vi "SRTS_Set Properties.vi"(8 "error in":errorcluster, 11 "TDMS in":refnum<class "TDMS.lvclass">) -> (0 "error out":errorcluster, 3 "TDMS out":refnum<class "TDMS.lvclass">)   [LabVIEW 2017, in "Report_lib.lvlib" / "TDMS.lvclass"]
uses:
  TDMS.lvclass
  Channels names.ctl
  TDMS.lvclass/TDMS.ctl
panel:
  out "size(s)":i32
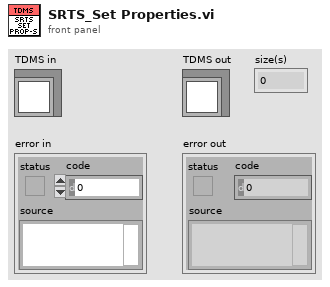
[diagram p1: front panel]
types:
  T1 = typedef "Channels names.ctl" = cluster{"AIM ch.names":string[], "TIM ch.names":string[], "RIM1 ch.names":string[], "RIM2 ch.names":string[], "RIM3 ch.names":string[], "AOM ch.names":string[], "DOM ch.hames":string[]}
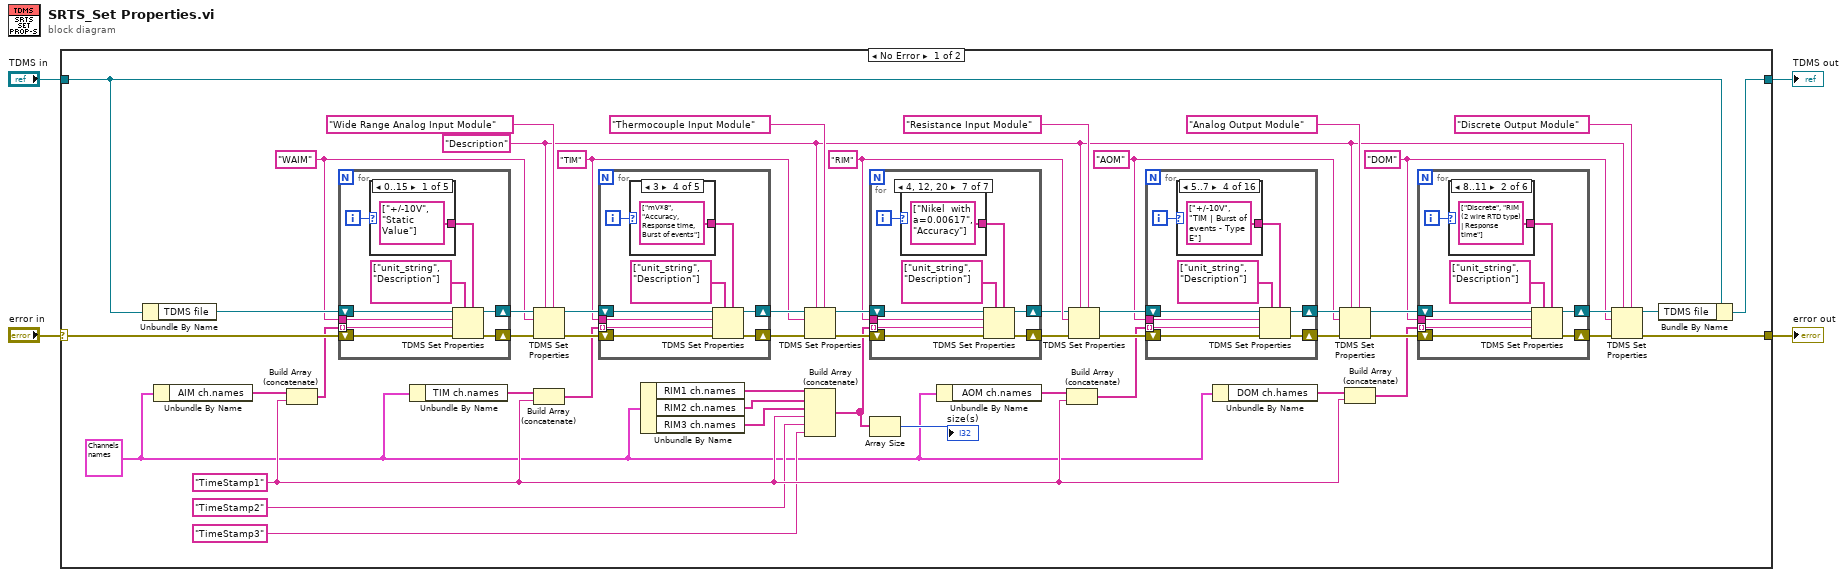
[diagram p0: block diagram]
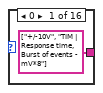
[diagram p2: hidden frame]
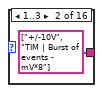
[diagram p3: hidden frame]
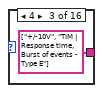
[diagram p4: hidden frame]
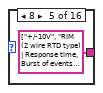
[diagram p5: hidden frame]
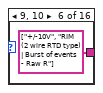
[diagram p6: hidden frame]
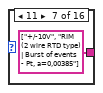
[diagram p7: hidden frame]
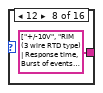
[diagram p8: hidden frame]
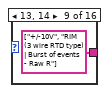
[diagram p9: hidden frame]
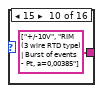
[diagram p10: hidden frame]
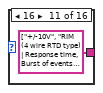
[diagram p11: hidden frame]
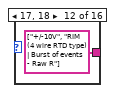
[diagram p12: hidden frame]
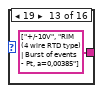
[diagram p13: hidden frame]
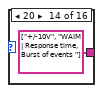
[diagram p14: hidden frame]
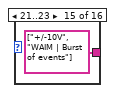
[diagram p15: hidden frame]
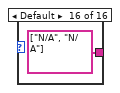
[diagram p16: hidden frame]
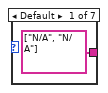
[diagram p17: hidden frame]
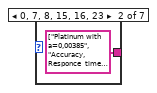
[diagram p18: hidden frame]
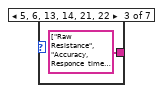
[diagram p19: hidden frame]
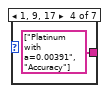
[diagram p20: hidden frame]
diagram:
  n1 = case shown="No Error" "error in" {
    selector: "error in" -> [w48 w142]
    tunnel: [w53 w142] -> w3
    tunnel: [w21 w141] -> w1
    tunnel: "TDMS in" -> [w22 w141]
    frame No Error {
      w5 = T1 {"AIM ch.names"=["05_waim_01ch", "05_waim_02ch", "05_waim_03ch", "05_waim_04ch", "05_waim_05ch", "05_waim_06ch", "05_waim_07ch", "05_waim_08ch", "05_waim_09ch", "05_waim_10ch", "05_waim_11ch", "05_waim_12ch", "05_waim_13ch", "05_waim_14ch", "05_waim_15ch", "05_waim_16ch", "05_waim_17ch", "05_waim_18ch", "05_waim_19ch", "05_waim_20ch", "05_waim_21ch", "05_waim_22ch", "05_waim_23ch", "05_waim_24ch", "05_waim_25ch", "05_waim_26ch", "05_waim_27ch", "05_waim_28ch", "05_waim_29ch", "05_waim_30ch", "05_waim_31ch", "05_waim_32ch", "01_tim_17ch", "01_tim_18ch", "01_tim_19ch", "01_tim_20ch", "01_tim_21ch", "01_tim_22ch", "01_tim_23ch", "01_tim_24ch", "01_tim_25ch", "01_tim_26ch", "01_tim_27ch", "01_tim_28ch", "01_tim_29ch", "01_tim_30ch", "01_tim_31ch", "01_tim_32ch"], "TIM ch.names"=["01_tim_01ch", "01_tim_02,14:16ch", "01_tim_03:09ch", "01_tim_10:13ch"], "RIM1 ch.names"=["02_rim_01ch", "02_rim_02ch", "02_rim_03ch", "02_rim_04ch", "02_rim_05ch", "02_rim_06ch", "02_rim_07ch", "02_rim_08ch", "reserve1"], "RIM2 ch.names"=["03_rim_01ch", "03_rim_02ch", "03_rim_03ch", "03_rim_04ch", "03_rim_05ch", "03_rim_06ch", "03_rim_07ch", "03_rim_08ch", "reserve2"], "RIM3 ch.names"=["04_rim_01ch", "04_rim_02ch", "04_rim_03ch", "04_rim_04ch", "04_rim_05ch", "04_rim_06ch", "04_rim_07ch", "04_rim_08ch", "reserve3"], "AOM ch.names"=["05_aom_01ch", "05_aom_02ch", "05_aom_03ch", "05_aom_04ch", "05_aom_05ch", "05_aom_06ch", "05_aom_07ch", "05_aom_08ch", "05_aom_09ch", "05_aom_10ch", "05_aom_11ch", "05_aom_12ch", "05_aom_13ch", "05_aom_14ch", "05_aom_15ch", "05_aom_16ch", "05_aom_17ch", "05_aom_18ch", "05_aom_19ch", "05_aom_20ch", "05_aom_21ch", "05_aom_22ch", "05_aom_23ch", "05_aom_24ch"], "DOM ch.hames"=["03_dom_01ch", "03_dom_02ch", "03_dom_03ch", "03_dom_04ch", "03_dom_05ch", "03_dom_06ch", "03_dom_07ch", "03_dom_08ch", "03_dom_09ch", "03_dom_10ch", "03_dom_11ch", "03_dom_12ch", "03_dom_13ch", "03_dom_14ch", "03_dom_15ch", "03_dom_16ch", "03_dom_17ch", "03_dom_18ch", "03_dom_19ch", "03_dom_20ch", "03_dom_21ch", "03_dom_22ch", "03_dom_23ch", "03_dom_24ch"]} ("Modules Channels names")
      w14 = "TimeStamp1"
      w24 = "DOM"
      w29 = "AOM"
      w36 = "RIM"
      w40 = "TIM"
      w50 = "Description"
      w45 = "WAIM"
      n2 = Unbundle By Name(w22) -> ("TDMS file"=w49:refnum<k34>)
      n3 = Unbundle By Name(w5) -> ("AIM ch.names"=w19:string[])
      n4 = Build Array (concatenate)(w19, w14) -> (w18:string[])
      n5 = for {
        tunnel: w18 -> [w120] mode=indexing
        tunnel: w45 -> [w119]
        shift-right: [w116] -> w46
        shift-left: w49 -> [w118]
        shift-right: [w115] -> w47
        shift-left: w48 -> [w117]
        i -> [w114]
        n6 = case shown="0..15" w114 {
          tunnel: [string[] ["+/-10V", "Static Value"] ("property names") string[] ["+/-10V", "Accuracy, Response time, Burst of events"] ("property names") string[] ["+/-10V", "Response time, Burst of events"] ("property names") string[] ["+/-10V", "Static Value"] ("property names") string[] ["N/A", "N/A"] ("property names")] -> w113
          frame 0..15 {
          }
          frame 16 {
          }
          frame 17..19 {
          }
          frame 20..47 {
          }
          frame Default {
          }
        }
        n7 = TDMS Set Properties(5:w113, 7:string[] ["unit_string", "Description"] ("property names"), 8:w117, 9:w120, 10:w119, 11:w118) -> (0:w115:errorcluster, 3:w116:refnum<k34>)  [unwired: 2 out]
      }
      n8 = Unbundle By Name(w5) -> ("TIM ch.names"=w20:string[])
      n9 = TDMS Set Properties(5:"Wide Range Analog Input Module", 7:w50, 8:w47, 10:w45, 11:w46) -> (0:w43:errorcluster, 3:w44:refnum<k34>)  [unwired: 1 in, 2 out]
      n10 = Build Array (concatenate)(w20, w14) -> (w39:string[])
      n11 = for {
        tunnel: w39 -> [w106] mode=indexing
        tunnel: w40 -> [w105]
        shift-right: [w102] -> w41
        shift-left: w44 -> [w104]
        shift-right: [w101] -> w42
        shift-left: w43 -> [w103]
        i -> [w100]
        n12 = case shown="3" w100 {
          tunnel: [string[] ["Type B, mV", "Accuracy"] ("property names") string[] ["Type E, mV", "Accuracy, Response time, Burst of events"] ("property names") string[] ["Type J,K,N,R,S,T,mV*32 mV", "Accuracy"] ("property names") string[] ["mV*8", "Accuracy, Response time, Burst of events"] ("property names") string[] ["N/A", "N/A"] ("property names")] -> w99
          frame 0 {
          }
          frame 1 {
          }
          frame 2 {
          }
          frame 3 {
          }
          frame Default {
          }
        }
        n13 = TDMS Set Properties(5:w99, 7:string[] ["unit_string", "Description"] ("property names"), 8:w103, 9:w106, 10:w105, 11:w104) -> (0:w101:errorcluster, 3:w102:refnum<k34>)  [unwired: 2 out]
      }
      n14 = Unbundle By Name(w5) -> ("RIM1 ch.names"=w10:string[], "RIM2 ch.names"=w9:string[], "RIM3 ch.names"=w8:string[])
      n15 = TDMS Set Properties(5:"Thermocouple Input Module", 7:w50, 8:w42, 10:w40, 11:w41) -> (0:w38:errorcluster, 3:w37:refnum<k34>)  [unwired: 1 in, 2 out]
      n16 = Build Array (concatenate)(w10, w9, w8, w14, "TimeStamp2", "TimeStamp3") -> (w12:string[])
      n17 = for {
        tunnel: w12 -> [w90] mode=indexing
        tunnel: w36 -> [w89]
        shift-right: [w86] -> w35
        shift-left: w37 -> [w88]
        shift-right: [w85] -> w34
        shift-left: w38 -> [w87]
        i -> [w84]
        n18 = case shown="4, 12, 20" w84 {
          tunnel: [string[] ["N/A", "N/A"] ("property names") string[] ["Platinum with a=0,00385", "Accuracy, Responce  time, Burst of events"] ("property names") string[] ["Raw Resistance", "Accuracy, Responce  time, Burst of events"] ("property names") string[] ["Platinum with a=0.00391", "Accuracy"] ("property names") string[] ["Copper  with a=0.00428", "Accuracy"] ("property names") string[] ["Copper  with a=0.00426", "Accuracy"] ("property names") string[] ["Nikel  with a=0.00617", "Accuracy"] ("property names")] -> w83
          frame Default {
          }
          frame 0, 7, 8, 15, 16, 23 {
          }
          frame 5, 6, 13, 14, 21, 22 {
          }
          frame 1, 9, 17 {
          }
          frame 2, 10, 18 {
          }
          frame 3, 11, 19 {
          }
          frame 4, 12, 20 {
          }
        }
        n19 = TDMS Set Properties(5:w83, 7:string[] ["unit_string", "Description"] ("property names"), 8:w87, 9:w90, 10:w89, 11:w88) -> (0:w85:errorcluster, 3:w86:refnum<k34>)  [unwired: 2 out]
      }
      n20 = Array Size(array=w12) -> (size(s)=→"size(s)":i32)
      n21 = Unbundle By Name(w5) -> ("AOM ch.names"=w17:string[])
      n22 = Build Array (concatenate)(w17, w14) -> (w16:string[])
      n23 = TDMS Set Properties(5:"Resistance Input Module", 7:w50, 8:w34, 10:w36, 11:w35) -> (0:w32:errorcluster, 3:w33:refnum<k34>)  [unwired: 1 in, 2 out]
      n24 = for {
        tunnel: w16 -> [w65] mode=indexing
        tunnel: w29 -> [w64]
        shift-right: [w61] -> w31
        shift-left: w33 -> [w63]
        shift-right: [w60] -> w30
        shift-left: w32 -> [w62]
        i -> [w59]
        n25 = case shown="5..7" w59 {
          tunnel: [string[] ["+/-10V", "TIM | Response time, Burst of events - mV*8"] ("property names") string[] ["+/-10V", "TIM | Burst of events - mV*8"] ("property names") string[] ["+/-10V", "TIM | Response time, Burst of events - Type E"] ("property names") string[] ["+/-10V", "TIM | Burst of events - Type E"] ("property names") string[] ["+/-10V", "RIM (2 wire RTD type) | Response time,  Burst of events - Pt, a=0,00385"] ("property names") string[] ["+/-10V", "RIM (2 wire RTD type) | Burst of events - Raw R"] ("property names") string[] ["+/-10V", "RIM (2 wire RTD type) | Burst of events - Pt, a=0,00385"] ("property names") string[] ["+/-10V", "RIM (3 wire RTD type) | Response time,  Burst of events - Pt, a=0,00385"] ("property names") string[] ["+/-10V", "RIM (3 wire RTD type) | Burst of events - Raw R"] ("property names") string[] ["+/-10V", "RIM (3 wire RTD type) | Burst of events - Pt, a=0,00385"] ("property names") string[] ["+/-10V", "RIM (4 wire RTD type) | Response time,  Burst of events - Pt, a=0,00385"] ("property names") string[] ["+/-10V", "RIM (4 wire RTD type) | Burst of events - Raw R"] ("property names") string[] ["+/-10V", "RIM (4 wire RTD type) | Burst of events - Pt, a=0,00385"] ("property names") string[] ["+/-10V", "WAIM | Response time, Burst of events "] ("property names") string[] ["+/-10V", "WAIM | Burst of events"] ("property names") string[] ["N/A", "N/A"] ("property names")] -> w58
          frame 0 {
          }
          frame 1..3 {
          }
          frame 4 {
          }
          frame 5..7 {
          }
          frame 8 {
          }
          frame 9, 10 {
          }
          frame 11 {
          }
          frame 12 {
          }
          frame 13, 14 {
          }
          frame 15 {
          }
          frame 16 {
          }
          frame 17, 18 {
          }
          frame 19 {
          }
          frame 20 {
          }
          frame 21..23 {
          }
          frame Default {
          }
        }
        n26 = TDMS Set Properties(5:w58, 7:string[] ["unit_string", "Description"] ("property names"), 8:w62, 9:w65, 10:w64, 11:w63) -> (0:w60:errorcluster, 3:w61:refnum<k34>)  [unwired: 2 out]
      }
      n27 = Unbundle By Name(w5) -> ("DOM ch.hames"=w15:string[])
      n28 = TDMS Set Properties(5:"Analog Output Module", 7:w50, 8:w30, 10:w29, 11:w31) -> (0:w28:errorcluster, 3:w27:refnum<k34>)  [unwired: 1 in, 2 out]
      n29 = Build Array (concatenate)(w15, w14) -> (w13:string[])
      n30 = for {
        tunnel: w13 -> [w134] mode=indexing
        tunnel: w24 -> [w133]
        shift-right: [w130] -> w26
        shift-left: w27 -> [w132]
        shift-right: [w129] -> w25
        shift-left: w28 -> [w131]
        i -> [w128]
        n31 = case shown="8..11" w128 {
          tunnel: [string[] ["Discrete", "TIM | Response time"] ("property names") string[] ["Discrete", "RIM (2 wire RTD type) | Response time"] ("property names") string[] ["Discrete", "RIM (3 wire RTD type) | Response time"] ("property names") string[] ["Discrete", "RIM (4 wire RTD type) | Response time"] ("property names") string[] ["Discrete", "WAIM | Response time"] ("property names") string[] ["N/A", "N/A"] ("property names")] -> w127
          frame 0..7 {
          }
          frame 8..11 {
          }
          frame 12..15 {
          }
          frame 16..19 {
          }
          frame 20..23 {
          }
          frame Default {
          }
        }
        n32 = TDMS Set Properties(5:w127, 7:string[] ["unit_string", "Description"] ("property names"), 8:w131, 9:w134, 10:w133, 11:w132) -> (0:w129:errorcluster, 3:w130:refnum<k34>)  [unwired: 2 out]
      }
      n33 = TDMS Set Properties(5:"Discrete Output Module", 7:w50, 8:w25, 10:w24, 11:w26) -> (0:w53:errorcluster, 3:w23:refnum<k34>)  [unwired: 1 in, 2 out]
      n34 = Bundle By Name(cluster=w22, "TDMS file"=w23) -> (w21:refnum<class "TDMS.lvclass">)
    }
    frame Error {
    }
  }
  "error out" <- w3
  "TDMS out" <- w1
